vi "QTM2SI.vi"(1 "Array":dbl[](array[numeric])) -> (14 "x":dbl, 15 "y":dbl, 16 "z":dbl, 17 "phi":dbl, 18 "theta":dbl, 19 "psi":dbl)   [LabVIEW 2014]
uses:
  <vilib>/imath/engines/lvmath2/RunTimeEngine/NodeEndStatement/NIMS_NodeEndStatement_Output.vi
  <instcachedir>/0/NIMS_NodeEndStatement_Output_53EC0D466D134D7ABD903AC30B43404B.lvgen/NIMS_NodeEndStatement_Output_53EC0D466D134D7ABD903AC30B43404B_005.vi
  <vilib>/imath/engines/lvmath2/RunTimeEngine/ErrorHandling/NIMS_Finalize Error.vi
  <instcachedir>/0/NIMS_NodeEndStatement_Output_53EC0D466D134D7ABD903AC30B43404B.lvgen/NIMS_NodeEndStatement_Output_53EC0D466D134D7ABD903AC30B43404B_001.vi
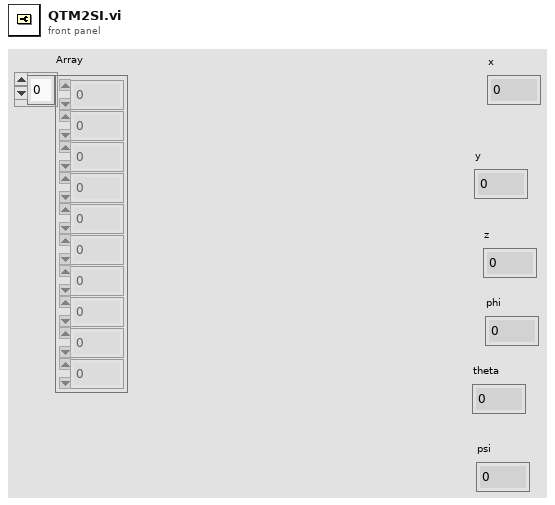
[diagram p1: front panel]
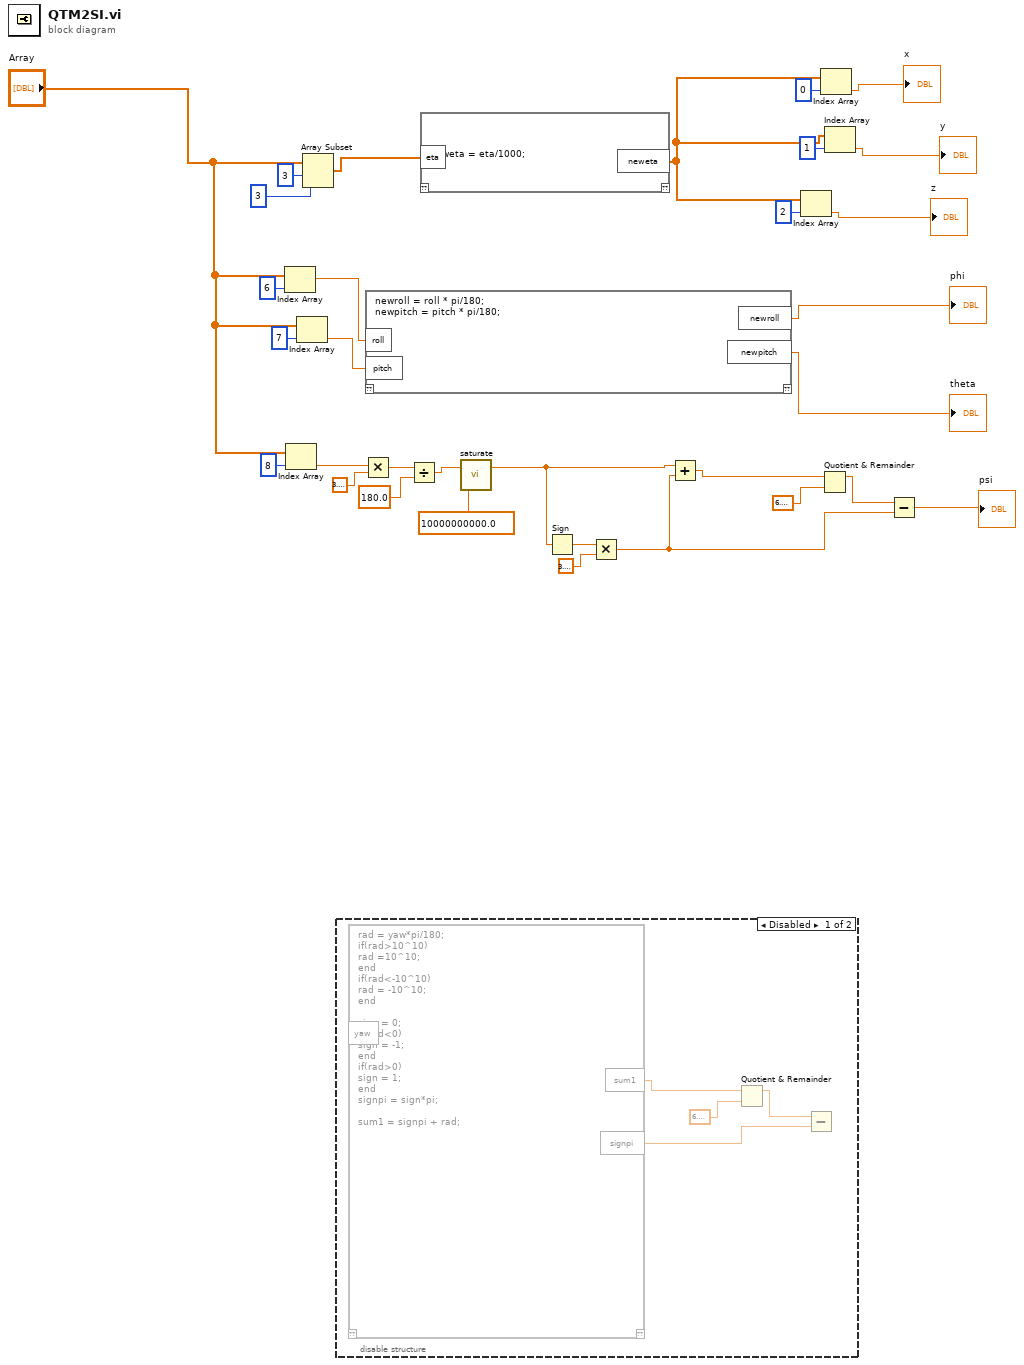
[diagram p0: block diagram]
diagram:
  n1 = Index Array(array="Array", index=6) -> (element=w25:dbl)
  n2 = Index Array(array="Array", index=8) -> (element=w12:dbl)
  n3 = Index Array(array="Array", index=7) -> (element=w24:dbl)
  n4 = Array Subset(array="Array", index=3, length=3) -> (w27:dbl[])
  n5 = disable-structure shown="Disabled" {
    frame Disabled {
      n6 = mathscript code="rad = yaw*pi/180;\nif(rad>10^10)\nrad =10^10;\nend\nif(rad<-10^10)\nrad = -10^10;\nend\n\nsign = 0;\nif(rad<0)\nsign = -1;\nend\nif(rad>0)\nsign = 1;\nend\nsignpi = sign*pi;\n\nsum1 = signpi + rad;"() -> ("signpi"=w34:dbl, "sum1"=w36:dbl)  [unwired: 2 in, 1 out]
      n7 = Quotient & Remainder(x=w36, y=6.283185307179586) -> (x-y*floor(x/y)=w33:dbl)  [unwired: 1 out]
      n8 = Subtract(x=w33, y=w34) -> ()  [unwired: 1 out]
    }
    frame Enabled {
    }
  }
  n9 = Multiply(x=w12, y=3.141592653589793) -> (x*y=w11:dbl)
  n10 = mathscript code="newroll = roll * pi/180;\nnewpitch = pitch * pi/180;"("roll"=w25, "pitch"=w24) -> ("newroll"=→"phi":dbl, "newpitch"=→"theta":dbl)  [unwired: 1 in, 1 out]
  n11 = Divide(x=w11, y=180.0) -> (x/y=w9:dbl)
  n12 = mathscript code="neweta = eta/1000;"("eta"=w27) -> ("neweta"=w23:dbl[])  [unwired: 1 in, 1 out]
  n13 = call "saturate.vi"("amplitude"=10000000000.0, "value"=w9) -> ("saturated"=w6:dbl)  [unwired: 1 out]
  n14 = Sign(1:w6) -> (0:w8:dbl)
  n15 = Multiply(x=w8, y=3.141592653589793) -> (x*y=w2:dbl)
  n16 = Add(x=w6, y=w2) -> (x+y=w3:dbl)
  n17 = Index Array(array=w23, index=2) -> (element=→"z":dbl)
  n18 = Quotient & Remainder(x=w3, y=6.283185307179586) -> (x-y*floor(x/y)=w4:dbl)  [unwired: 1 out]
  n19 = Index Array(array=w23, index=0) -> (element=→"x":dbl)
  n20 = Index Array(array=w23, index=1) -> (element=→"y":dbl)
  n21 = Subtract(x=w4, y=w2) -> (x-y=→"psi":dbl)
